vi "Start Insecure TCP.vi"(8 "error in (no error)":errorcluster, 11 "Server in":refnum<class "Server.lvclass">) -> (0 "error out":errorcluster, 3 "Server out":refnum<class "Server.lvclass">)   [LabVIEW 2020, in "HTTP Server.lvlib" / "Server.lvclass"]
uses:
  Server.lvclass
  Server.lvclass/Server.ctl
  lv-uri/URI/URI/URI.lvclass
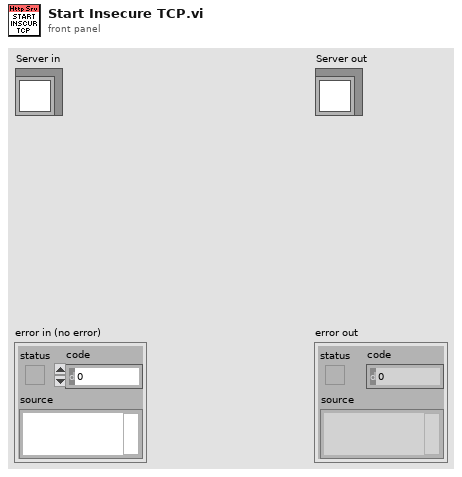
[diagram p1: front panel]
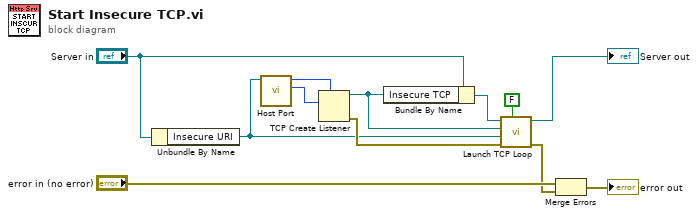
[diagram p0: block diagram]
diagram:
  n1 = Unbundle By Name("Server in") -> ("Insecure URI"=w5:refnum<class "URI.lvclass">)
  n2 = call "Host Port.vi"("URI in"=w5) -> ("Port"=w8:u16, "Host"=w9:u32)  [unwired: 8 in, 1 out]
  n3 = TCP Create Listener(7:w9, 10:w8) -> (0:w12:errorcluster, 3:w6:refnum<k5>)  [unwired: 3 in, 1 out]
  n4 = Bundle By Name(cluster="Server in", "Insecure TCP"=w6) -> (w2:refnum<class "Server.lvclass">)
  n5 = call "Launch TCP Loop.vi"("Secure"=FALSE, "error in (no error)"=w12, "Server URI"=w5, "TCP"=w6, "Server in"=w2) -> ("error out"=w3:errorcluster, "Server out"=→"Server out":refnum<class "Server.lvclass">)  [unwired: 5 in]
  n6 = Merge Errors("error in (no error)", w3) -> (→"error out":errorcluster)
